vi "set_ref.vi"(5 "ref in":refnum<class "RequestBuilder.lvclass">, 8 "error in (no error)":errorcluster, 11 "ref":u64) -> (0 "error out":errorcluster, 3 "ref out":refnum<class "RequestBuilder.lvclass">)   [LabVIEW 2020, in "reqwest.lvlib" / "RequestBuilder.lvclass"]
uses:
  RequestBuilder.lvclass
  RequestBuilder.lvclass/RequestBuilder.ctl
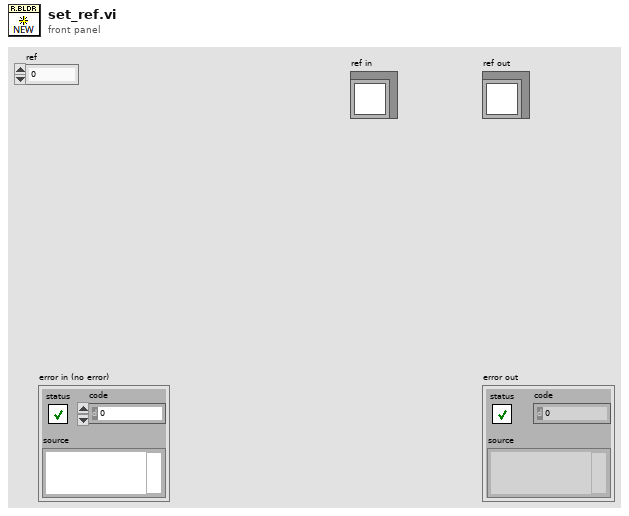
[diagram p1: front panel]
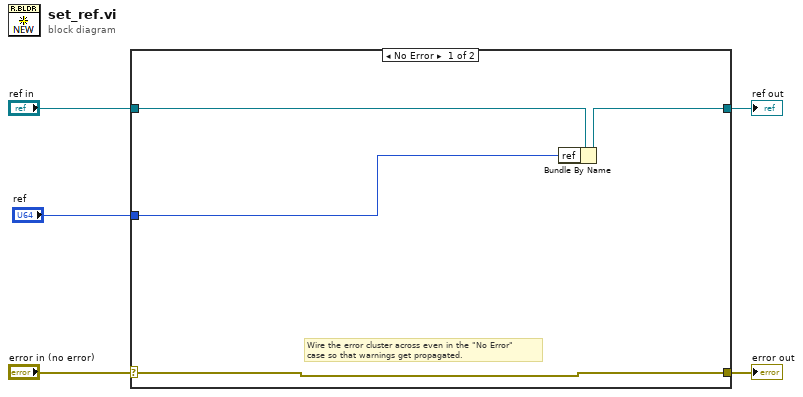
[diagram p0: block diagram]
diagram:
  n1 = case shown="No Error" "error in (no error)" {
    selector: "error in (no error)" -> [w8 w11]
    tunnel: [w8 w11] -> w4
    tunnel: [w7 w10] -> w2
    tunnel: "ref in" -> [w9 w10]
    tunnel: "ref" -> [w6 _]
    frame No Error {
      # "Wire the error cluster across even in the \"No Error\"\ncase so that warnings get propagated."
      n2 = Bundle By Name(cluster=w9, "ref"=w6) -> (w7:refnum<class "RequestBuilder.lvclass">)
    }
    frame Error {
    }
  }
  "error out" <- w4
  "ref out" <- w2
